vi "Result Last Step Output Meter Reading.vi"(8 "error in (no error)":errorcluster, 11 "VISA resource name":refnum<visa-resource-name>) -> (0 "error out":errorcluster, 2 "Result":string, 3 "VISA resource name out":refnum<visa-resource-name>)   [LabVIEW 2025, in "Chroma 19572.lvlib"]
uses:
  <instrlib>/Chroma 19572/Chroma 19572.lvlib
panel:
  # "Last Step Output Meter Reading"
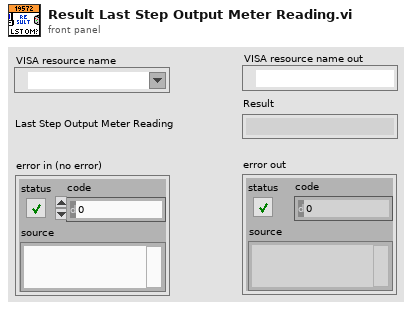
[diagram p1: front panel]
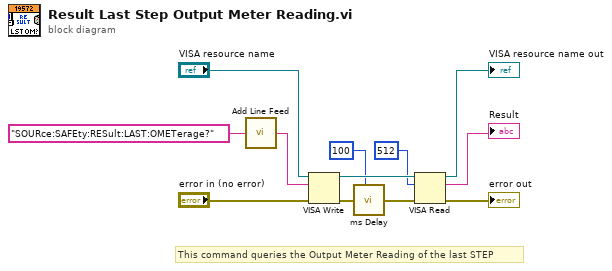
[diagram p0: block diagram]
diagram:
  # "This command queries the Output Meter Reading of the last STEP"
  n1 = call <instrlib>:"Add Line Feed.vi"("Command string"="SOURce:SAFEty:RESult:LAST:OMETerage?") -> ("Concatenated string"=w8:string)  [unwired: 4 in]
  n2 = VISA Write(VISA resource name="VISA resource name", write buffer=w8, error in (no error)="error in (no error)") -> (VISA resource name out=w10:refnum<visa-resource-name>, error out=w5:errorcluster)  [unwired: 1 out]
  n3 = call <instrlib>:"ms Delay.vi"("miliseconds to wait"=u32 100, "error in (no error)"=w5) -> ("error out"=w4:errorcluster)  [unwired: 6 in, 1 out]
  n4 = VISA Read(VISA resource name=w10, byte count=u32 512, error in (no error)=w4) -> (VISA resource name out=→"VISA resource name out":refnum<visa-resource-name>, read buffer=→"Result":string, error out=→"error out":errorcluster)  [unwired: 1 out]
